vi "Master Controller_Create.vi"(0 "reference in":refnum<class "Master Controller.lvclass">, 5 "error in (no error)":errorcluster) -> (14 "reference out":refnum<class "Master Controller.lvclass">, 19 "error out":errorcluster)   [LabVIEW 2015, in "Master Controller.lvclass"]
doc: "Constructor."
uses:
  Master Controller.lvclass
  <vilib>/addons/_AddQ/G#Object/G#Object.lvclass
  File Controller_llb/File Controller.lvclass
  GUI/GUI Controller_llb/GUI Controller.lvclass
  Subject Controller_llb/Subject Controller.lvclass
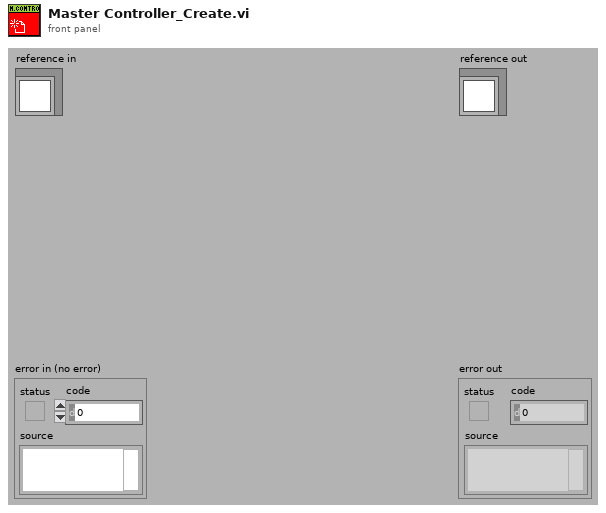
[diagram p1: front panel]
types:
  T1 = typedef "Master Controller.lvclass/ObjectAttributesRef.ctl" = refnum<data-value>
  T2 = typedef "Master Controller.lvclass/ClassAttributesRef.ctl" = refnum<data-value>
  T3 = typedef "Master Controller.lvclass/ClassAttributes.ctl" = cluster{"Dummy":bool, "Master Controller_ref":refnum<class "Master Controller.lvclass">}
  T4 = typedef "Master Controller.lvclass/ObjectAttributes.ctl" = cluster{"MyAttribute":dbl, "gui_controller_ref":refnum<class "GUI Controller.lvclass">, "file_controller_ref":refnum<class "File Controller.lvclass">, "subject_controller_ref":refnum<class "Subject Controller.lvclass">}
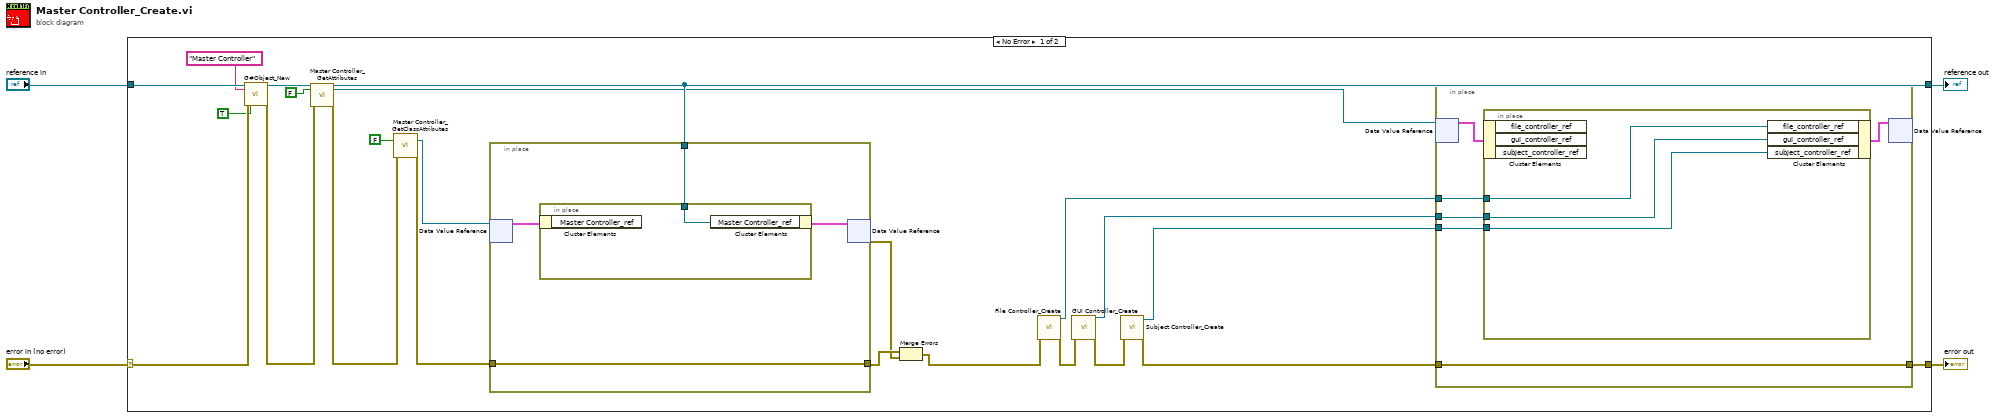
[diagram p0: block diagram]
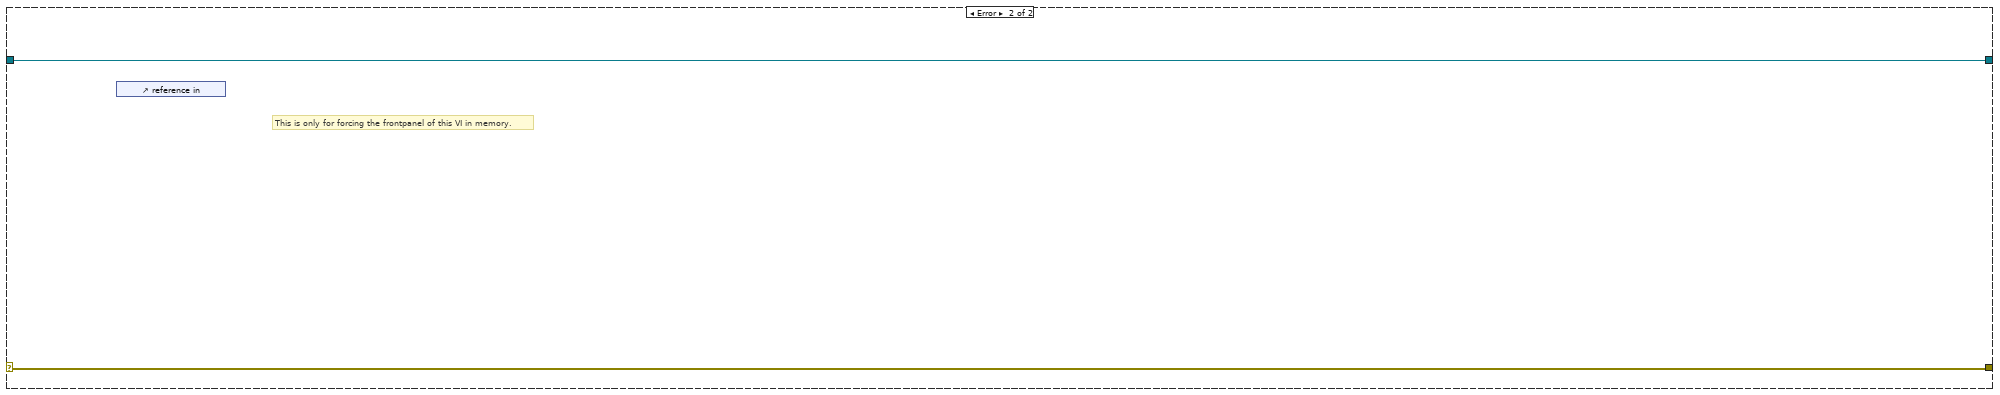
[diagram p2: hidden frame]
diagram:
  n1 = case shown="No Error" "error in (no error)" {
    selector: "error in (no error)" -> [w26 w43]
    tunnel: [w13 w43] -> w3
    tunnel: [w16 w42] -> w1
    tunnel: "reference in" -> [w27 w42]
    frame No Error {
      n2 = call <vilib>:"G#Object_New.vi"("reference in"=w27, "object name"="Master Controller", "error in (no error)"=w26, "user counter (T)?"=TRUE ("User Counter")) -> ("reference out"=w22:refnum<class "Master Controller.lvclass">, "error out"=w21:errorcluster)  [unwired: 13 in, 1 out]
      n3 = call "Master Controller_GetAttributes.vi"("reference in"=w22, "return data? (T)"=FALSE ("return data"), "error in (no error)"=w21) -> ("reference out"=w16:refnum<class "Master Controller.lvclass">, "attributes ref"=w12:T1, "error out"=w19:errorcluster)  [unwired: 13 in, 1 out]
      n4 = call "Master Controller_GetClassAttributes.vi"("return data? (T)"=FALSE, "error in (no error)"=w19) -> ("class attributes ref"=w17:T2, "error out"=w18:errorcluster)  [unwired: 14 in, 2 out]
      n5 = in-place {
        in-place-border: w18 -> [w38]
        in-place-border: [w38] -> w24
        in-place-border: w16 -> [w37]
        n6 = in-place-dvr #1(w17) -> (w39:T3)  [unwired: 1 out]
        n7 = in-place {
          in-place-border: w37 -> [w41]
          n8 = in-place-cluster #2(w39) -> ()  [unwired: 1 out]
          n9 = in-place-cluster #2("Master Controller_ref"=w41) -> (w40:T3)
        }
        n10 = in-place-dvr #1(w40) -> (w23:errorcluster)  [unwired: 1 out]
      }
      n11 = Merge Errors(w24, w23) -> (w11:errorcluster)
      n12 = call "File Controller_Create.vi"("error in (no error)"=w11) -> ("reference out"=w10:refnum<class "File Controller.lvclass">, "error out"=w9:errorcluster)  [unwired: 17 in]
      n13 = call "GUI Controller_Create.vi"("error in (no error)"=w9) -> ("reference out"=w8:refnum<class "GUI Controller.lvclass">, "error out"=w6:errorcluster)  [unwired: 17 in]
      n14 = call "Subject Controller_Create.vi"("error in (no error)"=w6) -> ("error out"=w5:errorcluster, "reference out"=w7:refnum<class "Subject Controller.lvclass">)  [unwired: 9 in]
      n15 = in-place {
        in-place-border: w5 -> [w31]
        in-place-border: [w31] -> w13
        in-place-border: w10 -> [w30]
        in-place-border: w8 -> [w29]
        in-place-border: w7 -> [w28]
        n16 = in-place-dvr #3(w12) -> (w32:T4)  [unwired: 1 out]
        n17 = in-place {
          in-place-border: w30 -> [w36]
          in-place-border: w29 -> [w35]
          in-place-border: w28 -> [w34]
          n18 = in-place-cluster #4(w32) -> ()  [unwired: 3 out]
          n19 = in-place-cluster #4("file_controller_ref"=w36, "gui_controller_ref"=w35, "subject_controller_ref"=w34) -> (w33:T4)
        }
        n20 = in-place-dvr #3(w33) -> ()  [unwired: 2 out]
      }
    }
    frame Error {
      # "This is only for forcing the frontpanel of this VI in memory."
      n21 = control-ref of="reference in"() -> ()  [unwired: 1 out]
    }
  }
  "error out" <- w3
  "reference out" <- w1
